vi "proxy messaging loop.vi"(9 "proxy queue":refnum<class "identifying queue.lvclass">, 10 "to this":refnum<class "identifying queue.lvclass">, 11 "to parent application":refnum<class "identifying queue.lvclass">) -> ()   [LabVIEW 2015, in "queue manager.lvclass"]
uses:
  queue manager.lvclass
  communicator queue/identifying queue.lvclass
  communicator queue/identifying queue.lvclass/identifying queue.ctl
  message/communicator message.lvclass/communicator message.ctl
  message/set sender.vi
  message/communicator message.lvclass
  communicator/communicator.lvclass
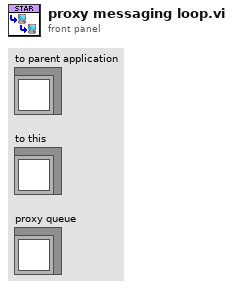
[diagram p1: front panel]
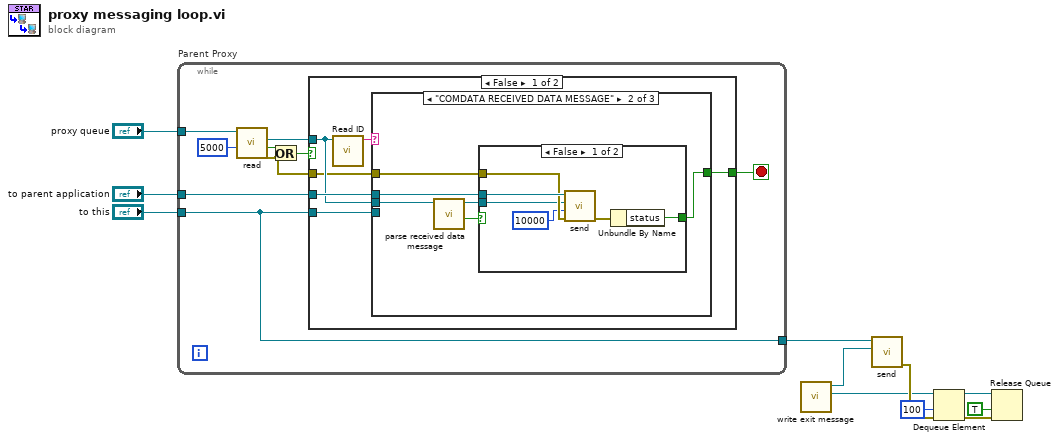
[diagram p0: block diagram]
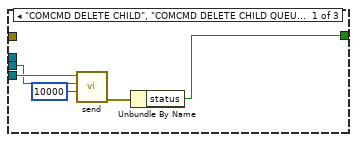
[diagram p2: hidden frame]
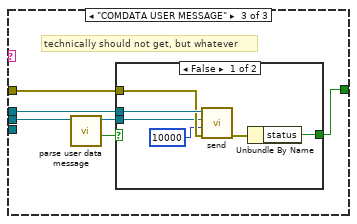
[diagram p4: hidden frame]
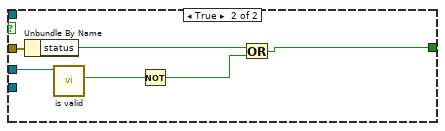
[diagram p6: hidden frame]
diagram:
  n1 = while "Parent Proxy" {
    tunnel: "proxy queue" -> [w19]
    tunnel: "to parent application" -> [w14]
    tunnel: "to this" -> [w12]
    tunnel: [w12] -> w8
    stop <- w16 stop-if-true
    n2 = call "read.vi"("timeout in ms (-1)"=5000, "identifying queue in"=w19) -> ("error out"=w17:errorcluster, "timed out?"=w20:bool, "message"=w15:refnum<class "communicator message.lvclass">)  [unwired: 7 in]
    n3 = Or(x=w20, y=w17) -> (x .or. y?=w18:bool)
    n4 = case shown="False" w18 {
      tunnel: w17 -> [w23 w61]
      tunnel: [w22 w58] -> w16
      tunnel: w15 -> [w24 _]
      tunnel: w14 -> [w25 w59]
      tunnel: w12 -> [w21 _]
      frame False {
        n5 = call "Read ID.vi"("communicator message in"=w24) -> ("ID"=w26:string)  [unwired: 10 in]
        n6 = case shown="\"COMDATA RECEIVED DATA MESSAGE\"" w26 {
          tunnel: w25 -> [_ w37 w49]
          tunnel: w24 -> [w29 w34 w46]
          tunnel: w23 -> [_ w36 w48]
          tunnel: [w28 w35 w47] -> w22
          tunnel: w21 -> [w30 _ _]
          frame "COMCMD DELETE CHILD", "COMCMD DELETE CHILD QUEUE", "COMCMD NEW CHILD", "COMCMD NEW CHILD QUEUE", "CONNDATA LOST CONNECTION", "CONNDATA NEW CONNECTION", Default {
            n7 = call "send.vi"("timeout in ms (-1)"=10000, "message"=w29, "message connection in"=w30) -> ("error out"=w31:errorcluster)  [unwired: 7 in, 1 out]
            n8 = Unbundle By Name(w31) -> ("status"=w28:bool)
          }
          frame "COMDATA RECEIVED DATA MESSAGE" {
            n9 = call "parse received data message.vi"("message"=w34) -> ("invalid?"=w32:bool, "data"=w33:refnum<class "communicator message.lvclass">)  [unwired: 9 in]
            n10 = case shown="False" w32 {
              tunnel: w37 -> [w43 _]
              tunnel: w36 -> [w42 _]
              tunnel: [w40 _] -> w35
              tunnel: w33 -> [w38 _]
              frame False {
                n11 = call "send.vi"("error in"=w42, "timeout in ms (-1)"=10000, "message"=w38, "message connection in"=w43) -> ("error out"=w41:errorcluster)  [unwired: 6 in, 1 out]
                n12 = Unbundle By Name(w41) -> ("status"=w40:bool)
              }
              frame True {
              }
            }
          }
          frame "COMDATA USER MESSAGE" {
            # "technically should not get, but whatever"
            n13 = call "parse user data message.vi"("message"=w46) -> ("invalid?"=w44:bool, "data"=w45:refnum<class "communicator message.lvclass">)  [unwired: 9 in]
            n14 = case shown="False" w44 {
              tunnel: w49 -> [w55 _]
              tunnel: w48 -> [w54 _]
              tunnel: [w52 _] -> w47
              tunnel: w45 -> [w50 _]
              frame False {
                n15 = call "send.vi"("error in"=w54, "timeout in ms (-1)"=10000, "message"=w50, "message connection in"=w55) -> ("error out"=w53:errorcluster)  [unwired: 6 in, 1 out]
                n16 = Unbundle By Name(w53) -> ("status"=w52:bool)
              }
              frame True {
              }
            }
          }
        }
      }
      frame True {
        n17 = Unbundle By Name(w61) -> ("status"=w60:bool)
        n18 = call "is valid.vi"("identifying queue in"=w59) -> ("valid?"=w57:bool)  [unwired: 9 in, 1 out]
        n19 = Not(x=w57) -> (.not. x?=w56:bool)
        n20 = Or(x=w60, y=w56) -> (x .or. y?=w58:bool)
      }
    }
  }
  n21 = call "write exit message.vi"() -> ("queue out"=w5:refnum<queue>, "message"=w7:refnum<class "communicator message.lvclass">)  [unwired: 10 in]
  n22 = call "send.vi"("message"=w7, "message connection in"=w8) -> ("error out"=w6:errorcluster)  [unwired: 8 in, 1 out]
  n23 = Dequeue Element(queue=w5, timeout in ms (-1)=100, error in (no error)=w6) -> (queue out=w3:refnum<queue>, error out=w4:errorcluster)  [unwired: 2 out]
  n24 = Release Queue(queue=w3, force destroy? (F)=TRUE, error in (no error)=w4) -> ()  [unwired: 3 out]
